vi "Read Data from Network Shared Variables.vi"(8 "error in":errorcluster, 10 "Page Configurations":T4(array[cluster]), 11 "Plot Data In":T1[][](array[typedef])) -> (0 "error out":errorcluster, 1 "Update Time":timestamp, 2 "New Data":bool, 3 "Plot Data Out":T1[][](array[typedef]))   [LabVIEW 2017, in "DTacq Plot Display Library.lvlib"]
uses:
  DTacq Plot Display Library.lvlib
  Plot Data--Cluster.ctl
  Network Shared Variables/Typedefs/X and Y Variant Arrays--Cluster.ctl
  Typedefs/Plot Channel Configruation--Cluster.ctl
  Network Shared Variables/Shared Variables Library.lvlib
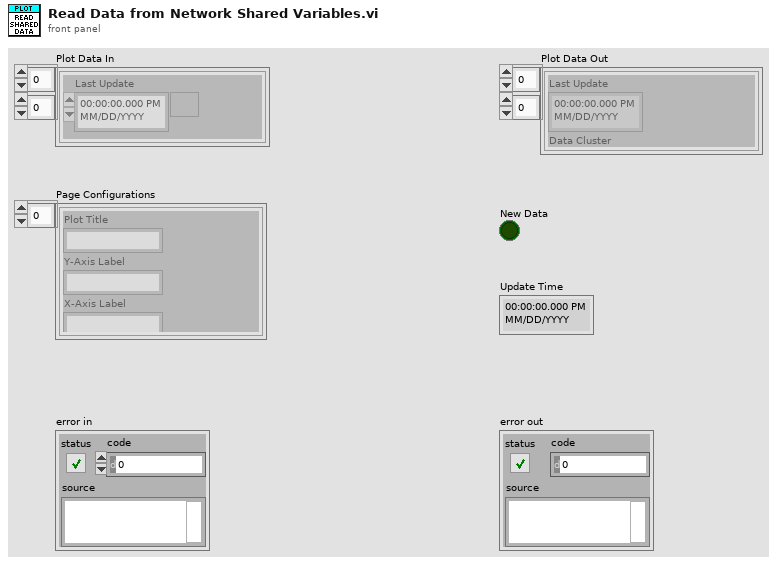
[diagram p1: front panel]
types:
  T1 = typedef "DTacq Plot Display Library.lvlib/Plot Data--Cluster.ctl" = cluster{"Last Update":timestamp, "Data Cluster":T2}
  T2 = typedef "Shared Variables Library.lvlib/X and Y Variant Arrays--Cluster.ctl" = cluster{"X-Data":variant[], "Y-Data":variant[]}
  T3 = typedef "DTacq Plot Display Library.lvlib/Plot Channel Configruation--Cluster.ctl" = cluster{"Shared Variable Reference":refnum<k21>, "Full Variable Name":string, "URL":string, "Descriptive Name":string, "Data Type":variant, "Colour":u32}
  T4 = cluster{"Plot Title":string, "Y-Axis Label":string, "X-Axis Label":string, "Plot Channel Configurations":T3[]}[]
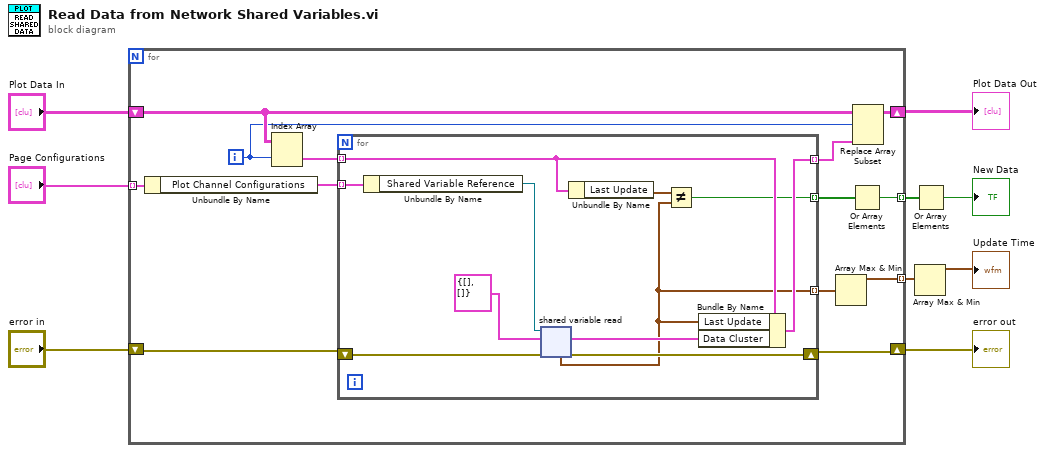
[diagram p0: block diagram]
diagram:
  n1 = for {
    tunnel: "Page Configurations" -> [w22] mode=indexing
    shift-right: [w19] -> w6
    shift-left: "error in" -> [w20]
    tunnel: [w17] -> w4 mode=indexing
    shift-right: [w14] -> w5
    shift-left: "Plot Data In" -> [w15]
    tunnel: [w10] -> w2 mode=indexing
    i -> [w13]
    n2 = Unbundle By Name(w22) -> ("Plot Channel Configurations"=w21:T3[])
    n3 = Index Array(array=w15, index (row)=w13) -> (element=w16:T1[])  [unwired: 1 in]
    n4 = for {
      tunnel: w21 -> [w33] mode=indexing
      shift-right: [w28] -> w19
      shift-left: w20 -> [w32]
      tunnel: [w24] -> w18 mode=indexing
      tunnel: w16 -> [w29] mode=indexing
      tunnel: [w26] -> w12 mode=indexing
      tunnel: [w23] -> w11 mode=indexing
      n5 = Unbundle By Name(w33) -> ("Shared Variable Reference"=w31:refnum<k21>)
      n6 = shared-variable-read(w31, w32, T2 {"X-Data"=[], "Y-Data"=[]} ("Data Cluster")) -> (w28:errorcluster, w27:T2, w23:timestamp)  [unwired: 1 out]
      n7 = Unbundle By Name(w29) -> ("Last Update"=w25:timestamp)
      n8 = Not Equal?(x=w25, y=w23) -> (x != y?=w24:bool)
      n9 = Bundle By Name(cluster=w29, "Last Update"=w23, "Data Cluster"=w27) -> (w26:T1)
    }
    n10 = Array Max & Min(array=w11) -> (max value=w10:timestamp)  [unwired: 3 out]
    n11 = Or Array Elements(Boolean array=w18) -> (logical OR=w17:bool)
    n12 = Replace Array Subset(array=w15, new element=w12, index (row)=w13) -> (w14:T1[][])  [unwired: 1 in]
  }
  "error out" <- w6
  "Plot Data Out" <- w5
  n13 = Array Max & Min(array=w2) -> (max value=→"Update Time":timestamp)  [unwired: 3 out]
  n14 = Or Array Elements(Boolean array=w4) -> (logical OR=→"New Data":bool)
